vi "Write Image delays.vi"(8 "error in (no error)":errorcluster, 10 "Image delays":string[](array[string]), 11 "Header in":refnum<class "Header.lvclass">) -> (0 "error out":errorcluster, 3 "Header out":refnum<class "Header.lvclass">)   [LabVIEW 2018, in "Header.lvclass"]
uses:
  Header.lvclass
  Header.lvclass/Header.ctl
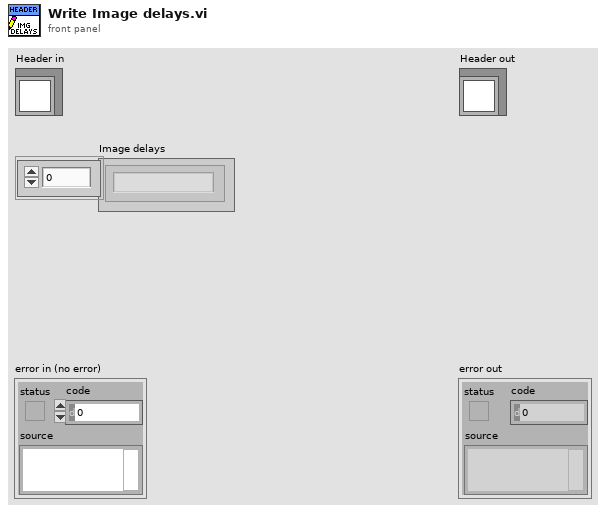
[diagram p1: front panel]
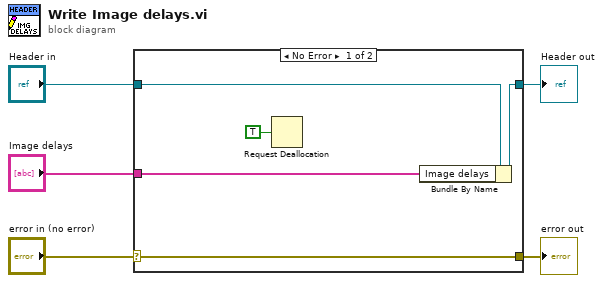
[diagram p0: block diagram]
diagram:
  n1 = case shown="No Error" "error in (no error)" {
    selector: "error in (no error)" -> [w10 w11]
    tunnel: [w10 w11] -> w4
    tunnel: [w8 w12] -> w2
    tunnel: "Header in" -> [w9 w12]
    tunnel: "Image delays" -> [w7 _]
    frame No Error {
      n2 = Request Deallocation(TRUE ("flag")) -> ()
      n3 = Bundle By Name(cluster=w9, "Image delays"=w7) -> (w8:refnum<class "Header.lvclass">)
    }
    frame Error {
    }
  }
  "error out" <- w4
  "Header out" <- w2
